vi "Close.vi"(8 "error in (no error)":errorcluster, 11 "GE 5565PIORC in":refnum<class "GE 5565PIORC.lvclass">) -> (0 "error out":errorcluster)   [LabVIEW 2016, in "GE 5565PIORC.lvclass"]
uses:
  GE 5565PIORC.lvclass
  GE 5565PIORC.lvclass/GE 5565PIORC.ctl
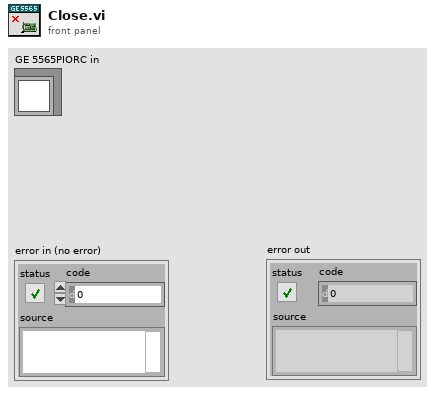
[diagram p1: front panel]
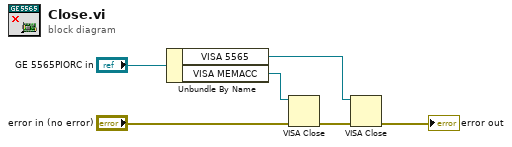
[diagram p0: block diagram]
diagram:
  n1 = Unbundle By Name("GE 5565PIORC in") -> ("VISA 5565"=w2:refnum<visa-resource-name>, "VISA MEMACC"=w4:refnum<visa-resource-name>)
  n2 = VISA Close(VISA resource name=w4, error in (no error)="error in (no error)") -> (error out=w3:errorcluster)
  n3 = VISA Close(VISA resource name=w2, error in (no error)=w3) -> (error out=→"error out":errorcluster)
